vi "strip cursor blink.vi"(8 "error in":errorcluster, 11 "input":string) -> (0 "error out":errorcluster, 3 "result string":string)   [LabVIEW 2018]
uses:
  <vilib>/regexp/Match Regular Expression.xnode
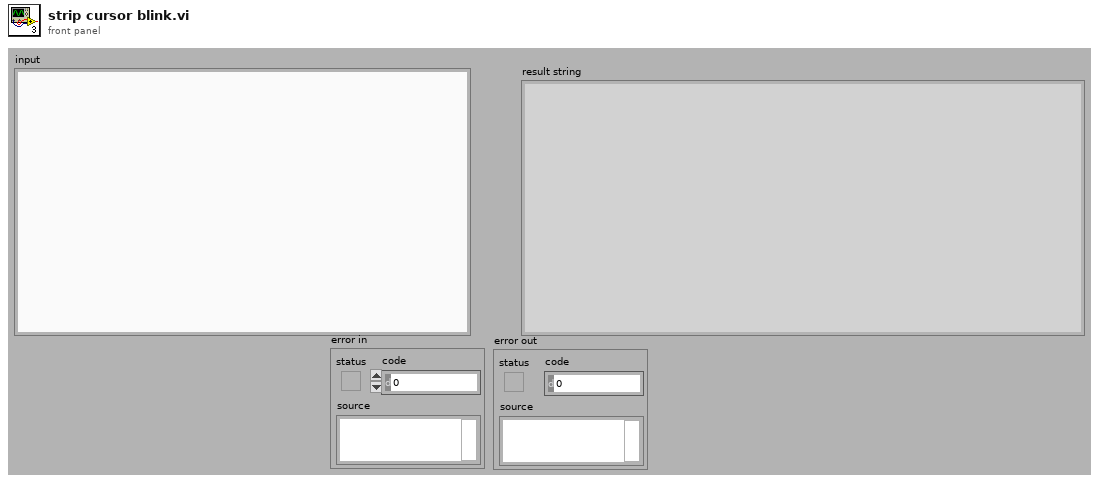
[diagram p1: front panel]
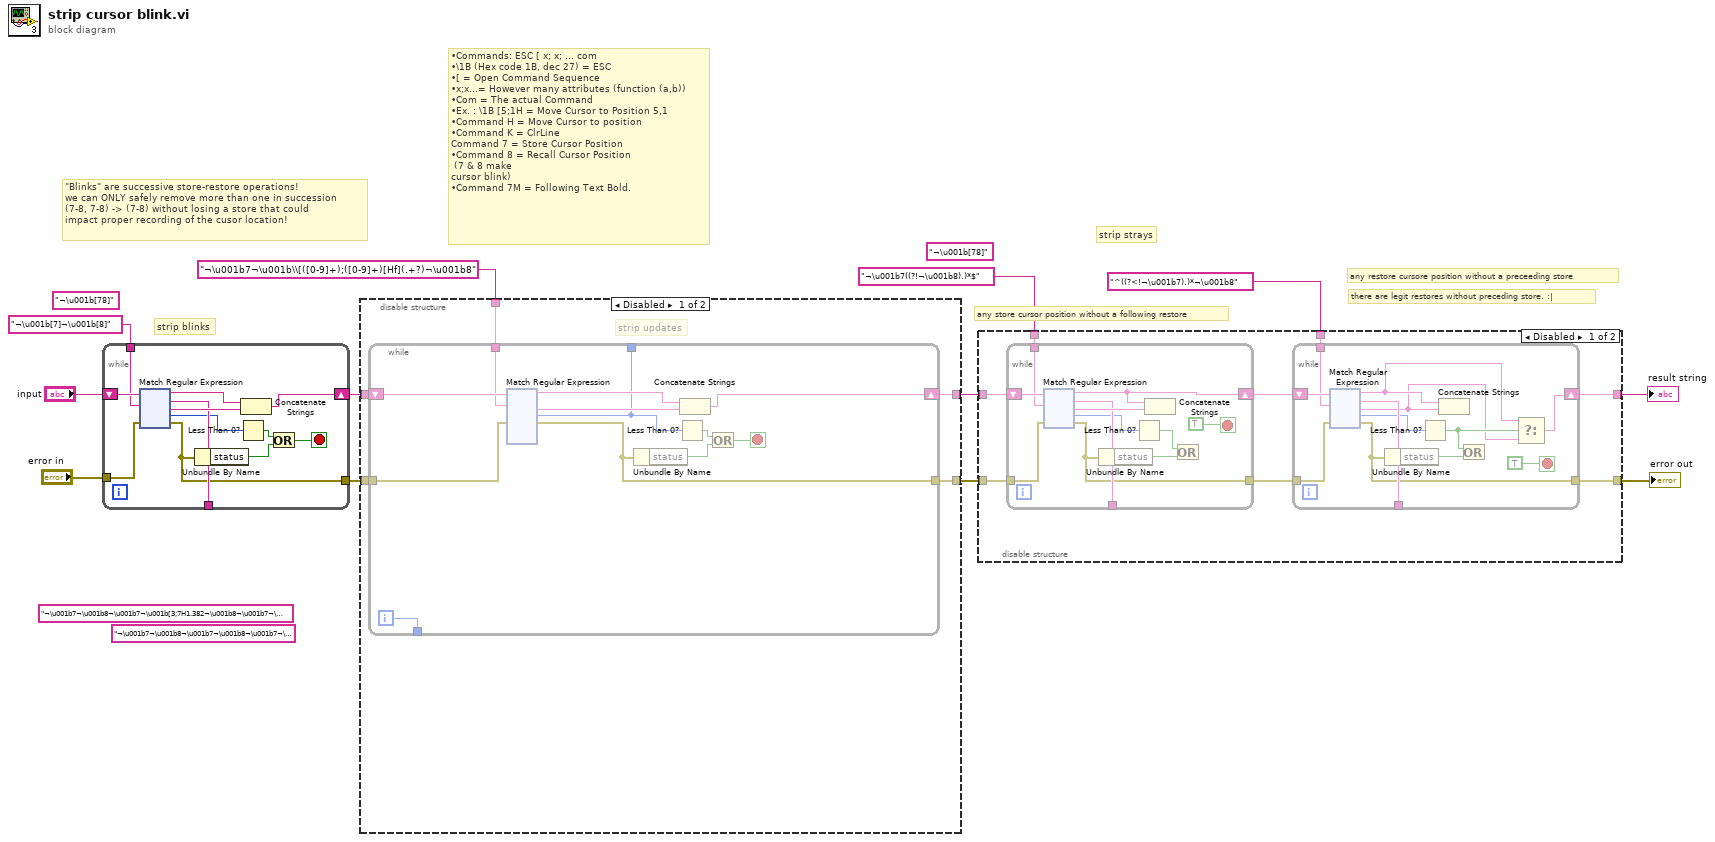
[diagram p0: block diagram]
diagram:
  (unwired) "¬\u001b[78]" ("search string")
  (unwired) "¬\u001b7¬\u001b8¬\u001b7¬\u001b[3;7H1.382¬\u001b8¬\u001b7¬\u001b8¬\u001b7¬\u001b8" ("string")
  (unwired) "¬\u001b[78]" ("search string")
  (unwired) "¬\u001b7¬\u001b8¬\u001b7¬\u001b8¬\u001b7¬\u001b8¬\u001b7¬\u001b8" ("string")
  # "•Commands: ESC [ x; x; … com \n•\\1B (Hex code 1B, dec 27) = ESC \n•[ = Open Command Sequence \n•x;x…= However many attributes (function (a,b)) \n•Com = The actual Command \n•Ex. : \\1B [5;1H = Move Cursor to Position 5,1 \n•Command H = Move Cursor to position \n•Command K = ClrLine\nCommand 7 = Store Cursor Position \n•Command 8 = Recall Cursor Position\n (7 & 8 make \ncursor blink) \n•Command 7M = Following Text Bold."
  # "\"Blinks\" are successive store-restore operations!\nwe can ONLY safely remove more than one in succession\n(7-8, 7-8) -> (7-8) without losing a store that could\nimpact proper recording of the cusor location!"
  # "there are legit restores without preceding store. :|"
  # "any restore cursore position without a preceeding store"
  # "any store cursor position without a following restore"
  # "strip blinks"
  # "strip strays"
  n1 = while {
    shift-right: [w22] -> w10
    shift-left: "input" -> [w20]
    tunnel: [w21] -> _
    tunnel: [w15] -> w7
    tunnel: "error in" -> [w14]
    tunnel: "¬\u001b[7]¬\u001b[8]" ("search string") -> [w13]
    stop <- w16 stop-if-true
    n2 = xnode "Match Regular Expression"("input string"=w20, "regular expression"=w13, "error in"=w14) -> ("before match"=w23:string, "whole match"=w21:string, "after match"=w24:string, "offset past match"=w19:i32, "error out"=w15:errorcluster)  [unwired: 3 in]
    n3 = Unbundle By Name(w15) -> ("status"=w17:bool)
    n4 = Less Than 0?(x=w19) -> (x < 0?=w18:bool)
    n5 = Concatenate Strings(w23, w24) -> (w22:string)
    n6 = Or(x=w18, y=w17) -> (x .or. y?=w16:bool)
  }
  n7 = disable-structure shown="Disabled" {
    disable-tunnel: "¬\u001b7¬\u001b\\[([0-9]+);([0-9]+)[Hf](.+?)¬\u001b8" ("search string") -> [w140 _]
    disable-tunnel: w10 -> [w139 w271]
    disable-tunnel: w7 -> [w138 w270]
    disable-tunnel: [w137 w271] -> w6
    disable-tunnel: [w136 w270] -> w5
    frame Disabled {
      # "strip updates"
      n8 = while {
        shift-right: [w150] -> w137
        shift-left: w139 -> [w149]
        tunnel: [w145] -> w136
        tunnel: w138 -> [w144]
        tunnel: w140 -> [w143]
        tunnel: [w142] -> _
        tunnel: [w141] -> _
        i -> [w141]
        stop <- w146 stop-if-true
        n9 = xnode "Match Regular Expression"("input string"=w149, "regular expression"=w143, "error in"=w144) -> ("before match"=w151:string, "after match"=w152:string, "offset past match"=w142:i32, "error out"=w145:errorcluster)  [unwired: 3 in, 3 out]
        n10 = Unbundle By Name(w145) -> ("status"=w147:bool)
        n11 = Less Than 0?(x=w142) -> (x < 0?=w148:bool)
        n12 = Concatenate Strings(w151, w152) -> (w150:string)
        n13 = Or(x=w148, y=w147) -> (x .or. y?=w146:bool)
      }
    }
    frame Enabled {
    }
  }
  n14 = disable-structure shown="Disabled" {
    disable-tunnel: "¬\u001b7((?!¬\u001b8).)*$" ("search string") -> [w279 _]
    disable-tunnel: w6 -> [w278 w526]
    disable-tunnel: w5 -> [w277 w525]
    disable-tunnel: [w274 w525] -> w4
    disable-tunnel: [w273 w526] -> w3
    disable-tunnel: "^((?<!¬\u001b7).)*¬\u001b8" ("search string") -> [w272 _]
    frame Disabled {
      n15 = while {
        shift-right: [w403] -> w276
        shift-left: w278 -> [w411]
        tunnel: [w412] -> _
        tunnel: [w407] -> w275
        tunnel: w277 -> [w406]
        tunnel: w279 -> [w405]
        stop <- TRUE stop-if-true
        n16 = xnode "Match Regular Expression"("input string"=w411, "regular expression"=w405, "error in"=w406) -> ("before match"=w403:string, "whole match"=w412:string, "after match"=w413:string, "offset past match"=w410:i32, "error out"=w407:errorcluster)  [unwired: 3 in]
        n17 = Unbundle By Name(w407) -> ("status"=w408:bool)
        n18 = Less Than 0?(x=w410) -> (x < 0?=w409:bool)
        n19 = Concatenate Strings(w403, w413) -> ()  [unwired: 1 out]
        n20 = Or(x=w409, y=w408) -> ()  [unwired: 1 out]
      }
      n21 = while {
        shift-right: [w280] -> w273
        shift-left: w276 -> [w290]
        tunnel: [w291] -> _
        tunnel: [w287] -> w274
        tunnel: w275 -> [w286]
        tunnel: w272 -> [w285]
        stop <- TRUE stop-if-true
        n22 = xnode "Match Regular Expression"("input string"=w290, "regular expression"=w285, "error in"=w286) -> ("before match"=w282:string, "whole match"=w291:string, "after match"=w281:string, "offset past match"=w289:i32, "error out"=w287:errorcluster)  [unwired: 3 in]
        n23 = Unbundle By Name(w287) -> ("status"=w288:bool)
        n24 = Less Than 0?(x=w289) -> (x < 0?=w283:bool)
        n25 = Concatenate Strings(w282, w281) -> ()  [unwired: 1 out]
        n26 = Or(x=w283, y=w288) -> ()  [unwired: 1 out]
        n27 = Select(t=w282, s=w283, f=w281) -> (s? t:f=w280:string)
      }
    }
    frame Enabled {
    }
  }
  "result string" <- w3
  "error out" <- w4
